vi "update last message.vi"(8 "error in (no error)":errorcluster, 11 "Server in":refnum<class "Server.lvclass">) -> (0 "error out":errorcluster, 3 "Server out":refnum<class "Server.lvclass">)   [LabVIEW 2018, in "Server.lvclass"]
uses:
  Server.lvclass
  Server.lvclass/Server.ctl
  RxTx/RxTx.lvclass
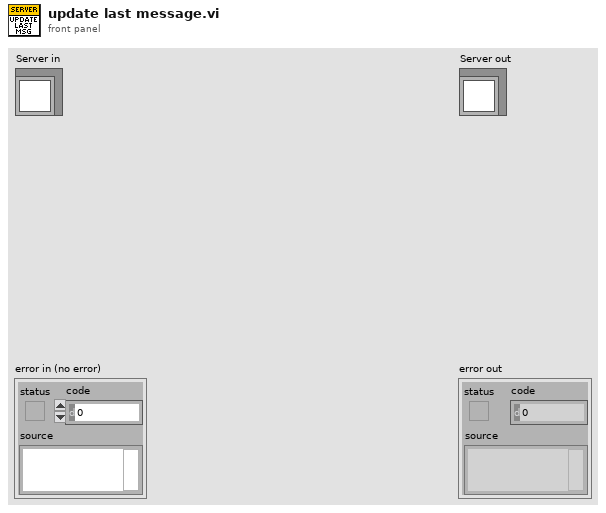
[diagram p1: front panel]
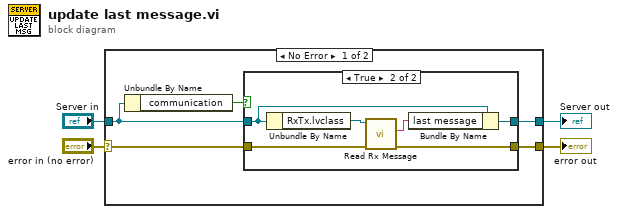
[diagram p0: block diagram]
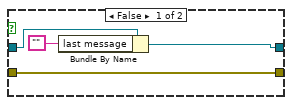
[diagram p2: hidden frame]
diagram:
  n1 = case shown="No Error" "error in (no error)" {
    selector: "error in (no error)" -> [w7 w21]
    tunnel: [w6 w21] -> w3
    tunnel: [w5 w20] -> w1
    tunnel: "Server in" -> [w8 w20]
    frame No Error {
      n2 = Unbundle By Name(w8) -> ("communication"=w9:bool)
      n3 = case shown="True" w9 {
        tunnel: w8 -> [w12 w16]
        tunnel: w7 -> [w13 w18]
        tunnel: [w13 w17] -> w6
        tunnel: [w11 w14] -> w5
        frame False {
          n4 = Bundle By Name(cluster=w12, "last message"="") -> (w11:refnum<class "Server.lvclass">)
        }
        frame True {
          n5 = Unbundle By Name(w16) -> ("RxTx.lvclass"=w19:refnum<class "RxTx.lvclass">)
          n6 = call "Read Rx Message.vi"("error in (no error)"=w18, "RxTx in"=w19) -> ("error out"=w17:errorcluster, "Rx Message"=w15:string)  [unwired: 7 in, 1 out]
          n7 = Bundle By Name(cluster=w16, "last message"=w15) -> (w14:refnum<class "Server.lvclass">)
        }
      }
    }
    frame Error {
    }
  }
  "error out" <- w3
  "Server out" <- w1
